vi "Package Version.vi"(8 "error in (no error)":errorcluster, 11 "GPack File in":refnum<class "GPack File.lvclass">) -> (0 "error out":errorcluster, 2 "Package Version":string)   [LabVIEW 2020, in "GPack.lvlib" / "GPack File.lvclass"]
uses:
  GPack File.lvclass
  GPack File.lvclass/GPack File.ctl
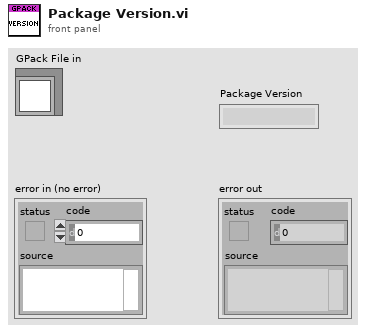
[diagram p1: front panel]
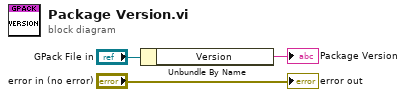
[diagram p0: block diagram]
diagram:
  n1 = Unbundle By Name("GPack File in") -> ("Version"=→"Package Version":string)
  "error out" <- "error in (no error)"
